vi "numpad.vi"(11 "Array":bool[](array[boolean])) -> (3 "Cluster":T1)   [LabVIEW 2019]
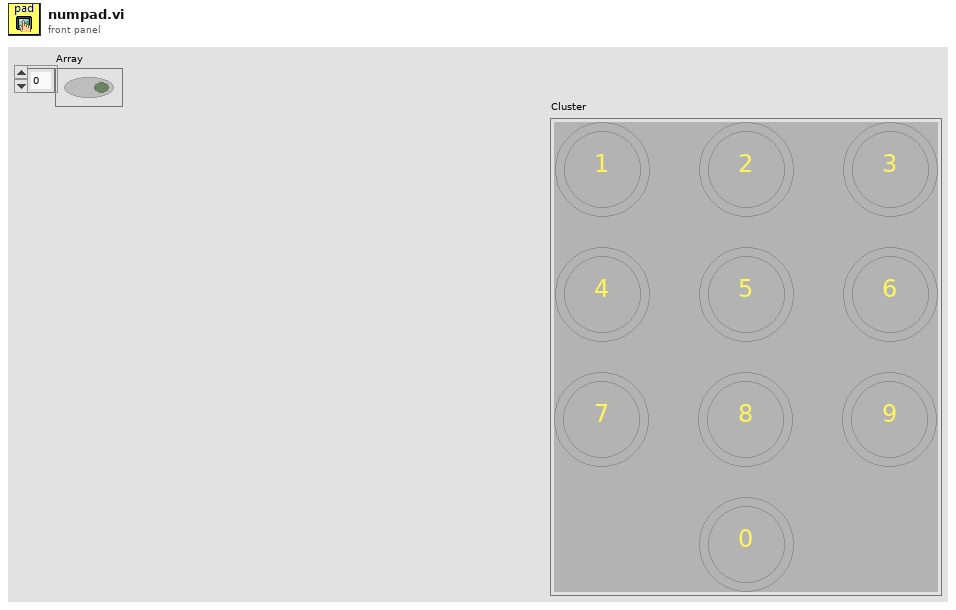
[diagram p1: front panel]
types:
  T1 = cluster{"Boolean 0":bool, "Boolean 9":bool, "Boolean 8":bool, "Boolean 7":bool, "Boolean 6":bool, "Boolean 5":bool, "Boolean 4":bool, "Boolean 3":bool, "Boolean 2":bool, "Boolean 1":bool}
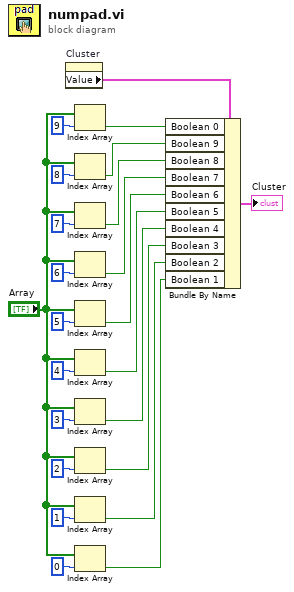
[diagram p0: block diagram]
diagram:
  n1 = property on="Cluster" class="Clust (strict)"() -> ("Value"=w22:T1)  [unwired: 2 in, 2 out]
  n2 = Index Array(array="Array", index=9) -> (element=w1:bool)
  n3 = Index Array(array="Array", index=8) -> (element=w2:bool)
  n4 = Index Array(array="Array", index=7) -> (element=w3:bool)
  n5 = Index Array(array="Array", index=6) -> (element=w4:bool)
  n6 = Index Array(array="Array", index=5) -> (element=w5:bool)
  n7 = Index Array(array="Array", index=4) -> (element=w6:bool)
  n8 = Index Array(array="Array", index=3) -> (element=w7:bool)
  n9 = Index Array(array="Array", index=2) -> (element=w8:bool)
  n10 = Index Array(array="Array", index=1) -> (element=w9:bool)
  n11 = Index Array(array="Array", index=0) -> (element=w10:bool)
  n12 = Bundle By Name(cluster=w22, "Boolean 0"=w1, "Boolean 9"=w2, "Boolean 8"=w3, "Boolean 7"=w4, "Boolean 6"=w5, "Boolean 5"=w6, "Boolean 4"=w7, "Boolean 3"=w8, "Boolean 2"=w9, "Boolean 1"=w10) -> (→"Cluster":T1)
